vi "HFRR ADV v026 new software.vi"() -> ()   [LabVIEW 2025] (continued)
            n898 = Number To Fractional String(number=w899, width (-)=i16 4, precision (6)=i16 7) -> (F-format string=w905:string)  [unwired: 1 in]
            n899 = Number To Fractional String(number=w901, width (-)=i16 10 ("precision (6)"), precision (6)=i16 7) -> (F-format string=w931:string)  [unwired: 1 in]
            n900 = Concatenate Strings("[CH1]" ("string"), w931, " - 5x Gain" ("string"), "\r") -> (w921:string)
            n901 = Concatenate Strings("[CH2]" ("string"), w922, " - 10x Gain" ("string"), "\r") -> (w920:string)
            n902 = Concatenate Strings("[CH3]" ("string"), w917, " - 20x Gain" ("string"), "\r") -> (w911:string)
            n903 = Concatenate Strings("[CH4]" ("string"), w905, " - 100x Gain" ("string"), "\r") -> (w904:string)
            n904 = String To Path(string="C:\\LAB-IQ\\Image Calibrate v01.dcf") -> (path=w934:path)
            n905 = Concatenate Strings(w921, w920, w911, w904) -> (w919:string)
            n906 = call <vilib>:"Write Characters To File.vi"("append to file? (new file:F)"=FALSE, "character string"=w919, "file path (dialog if empty)"=w934) -> ()  [unwired: 2 in, 1 out]
          }
          frame #2 {
            n907 = String To Path(string="C:\\LAB-IQ\\Image Calibrate v01.dcf") -> (path=w937:path)
            n908 = Open/Create/Replace File ("Open File")(file path (use dialog)=w937) -> (refnum out=w938:refnum<file>)  [unwired: 5 in, 2 out]
            n909 = for {
              N: 4 -> [_]
              tunnel: w938 -> [w944]
              i -> [w940]
              n910 = Read from Text File ("Read File")(file (use dialog)=w944) -> (text=w945:string)  [unwired: 3 in, 3 out]
              n911 = String Subset(string=w945, offset (0)=6, length (rest)=10 ("length (rest)")) -> (substring=w941:string)
              n912 = Fract/Exp String To Number(string=w941) -> (number=w939:dbl)  [unwired: 3 in, 1 out]
              n913 = case shown="3" w940 {
                tunnel: w939 -> [w946 w947 _ w948 _]
                frame 0 {
                  n914 = local write "5x Gain"(w946) -> ()
                }
                frame 1 {
                  n915 = local write "10x Gain"(w947) -> ()
                }
                frame 2 {
                }
                frame 3 {
                  n916 = local write "100x gain"(w948) -> ()
                }
                frame 4, Default {
                }
              }
            }
          }
          frame #3 {
            n917 = call "IMAGE ANALYSIS.vi"("Enum"=POST_ANALYSIS_ENUM."SHOW UI") -> ()  [unwired: 9 in, 2 out]
          }
          frame #4 {
            n918 = Not(x=w951) -> (.not. x?=w950:bool)
            n919 = local write "Save Change"(w950) -> ()
          }
        }
      }
    }
    n920 = case shown="False" w841 {
      tunnel: w840 -> [w867 _]
      frame False {
        n921 = case shown="True" w867 {
          frame False {
          }
          frame True {
            n922 = local read "Set Humidity:"() -> (w871:dbl)
            n923 = local read "Set Humidity:"() -> (w874:dbl)
            n924 = local read "Humidity ( %RH )"() -> (w875:dbl)
            n925 = Subtract(x=w871, y=2.0) -> (x-y=w869:dbl)
            n926 = Add(x=w874, y=2.0) -> (x+y=w870:dbl)
            n927 = In Range and Coerce(upper limit=w870, x=w875, lower limit=w869) -> (In Range?=w868:bool)  [unwired: 1 out]
            n928 = case shown="True" w868 {
              frame False {
              }
              frame True {
                n929 = case shown="True" "Manual Humididty Reached" {
                  selector: "Manual Humididty Reached" -> [_ w878]
                  frame False {
                  }
                  frame True {
                    n930 = Not(x=w878) -> (.not. x?=w877:bool)
                    n931 = local write "Manual Humididty Reached"(w877) -> ()
                    n932 = local read "EVENT LOG"() -> (w880:string)
                    n933 = call "Event Log.vi"("Content"="Target Humidity reached", "EVENT LOG"=w880) -> ("EVENT LOG"=w879:string)  [unwired: 8 in, 1 out]
                    n934 = local write "EVENT LOG"(w879) -> ()
                  }
                }
              }
            }
          }
        }
      }
      frame True {
        n935 = local write "Manual Humididty Reached"(TRUE ("Manual Humididty Reached")) -> ()
      }
    }
    n936 = local read "Cap Live Image"() -> (w861:bool)
    n937 = local read "SCAR MEASURMENT"() -> (w864:enum32{"Auto Scar", "Manual Scar"})
    n938 = Wait (ms)(milliseconds to wait=u32 250) -> ()  [unwired: 1 out]
    n939 = Equal?(x=w864, y=enum32{"Auto Scar", "Manual Scar"}."Manual Scar" ("SCAR MEASURMENT")) -> (x = y?=w862:bool)
    n940 = And(x=w862, y=w861) -> (x .and. y?=w860:bool)
    n941 = case shown="True" w860 {
      selector: w860 -> [_ w1176]
      frame False {
      }
      frame True {
        n942 = stacked-sequence {
          tunnel: [_ _ _ w1191 _] -> _
          tunnel: w1176 -> [_ _ _ _ w1198]
          frame #0 {
            w1177 = 0.0
            n943 = local write "Major Axis"(w1177) -> ()
            n944 = local write "Minor Axis"(w1177) -> ()
            n945 = local write "Average"(w1177) -> ()
          }
          frame #1 {
            n946 = call "CAMERA LIVE FEED FGV.vi"("Enum - Menu"=CAMERA_LIVE_FEED_ENUM."CAMERA MINIMIZE") -> ()  [unwired: 9 in, 2 out]
          }
          frame #2 {
            n947 = local read "FILE 3"() -> (w1185:string)
            n948 = call <vilib>:"Trim Whitespace.vi"("string"="C:\\LAB-IQ\\images\\") -> ("trimmed string"=w1187:string)  [unwired: 1 in]
            n949 = String To Path(string=w1187) -> (path=w1186:path)
            n950 = Concatenate Strings(w1185, ".png" ("string")) -> (w1184:string)
            n951 = Build Path(base path=w1186, name or relative path=w1184) -> (appended path=w1182:path)
            n952 = Path To String(path=w1182) -> (string=w1181:string)
            n953 = call "CAMERA LIVE FEED FGV.vi"("Enum - Menu"=CAMERA_LIVE_FEED_ENUM."CAMERA SAVE", "Image Path"=w1181) -> ("error out"=w1179:errorcluster)  [unwired: 8 in, 1 out]
            n954 = case shown="No Error" w1179 {
              frame No Error {
                n955 = One Button Dialog(message="Image saved successfully") -> ()  [unwired: 1 in, 1 out]
              }
              frame Error {
              }
            }
          }
          frame #3 {
            n956 = call "LIST FILE NAMES.vi"() -> ("error out"=w1193:errorcluster, "filenames"=w1190:string[])  [unwired: 10 in]
            n957 = call "IMAGE ANALYSIS.vi"("Enum"=POST_ANALYSIS_ENUM."SHOW UI", "error in"=w1193) -> ("error out"=w1191:errorcluster)  [unwired: 8 in, 1 out]
            n958 = property on="Test File List :" class="CmbBox"("Strings[]"=w1190) -> ()  [unwired: 2 in, 2 out]
          }
          frame #4 {
            (unwired) T23."Report" ("Main Dashboard Buttons")
            (unwired) T25."Report" ("Main Dashboard Buttons")
            n959 = Not(x=w1198) -> (.not. x?=w1197:bool)
            n960 = local write "Zoom Factore"(0.0 ("Zoom Factore")) -> ()
            n961 = local write "Cap Live Image"(w1197) -> ()
            n962 = local write "Main Tab"(T2."Adv Scar Report" ("Main Tab")) -> ()
            n963 = property on="Cap Live Image" class="Bool (strict)"("BoolText.Text"="Capture Image" ("Boolean Text.Text")) -> ()  [unwired: 2 in, 2 out]
            n964 = local write "Main Dashboard Buttons"(T1."Report" ("Main Dashboard Buttons")) -> ()
          }
        }
      }
    }
    n965 = local read "change Gain"() -> (w844:bool)
    n966 = local read "Back Square"() -> (w843:bool)
    n967 = case shown="True" w844 {
      selector: w844 -> [_ w888]
      frame False {
      }
      frame True {
        n968 = stacked-sequence {
          tunnel: w888 -> [_ w896]
          frame #0 {
            n969 = local read "Actual (µm)"() -> (w892:dbl)
            n970 = local read "Pixel Value"() -> (w891:dbl)
            n971 = local read "Magnification :"() -> (w890:string)
            n972 = Divide(x=w892, y=w891) -> (x/y=w889:dbl)
            n973 = case shown="\"10x\"" w890 {
              tunnel: w889 -> [w893 w894]
              frame "10x" {
                n974 = local write "10x Gain"(w893) -> ()
              }
              frame "5x", Default {
                n975 = local write "5x Gain"(w894) -> ()
              }
            }
          }
          frame #1 {
            n976 = Not(x=w896) -> (.not. x?=w895:bool)
            n977 = local write "change Gain"(w895) -> ()
          }
        }
      }
    }
    n978 = case shown="True" w843 {
      selector: w843 -> [_ w886]
      frame False {
      }
      frame True {
        n979 = Not(x=w886) -> (.not. x?=w885:bool)
        n980 = local write "Back Square"(w885) -> ()
        n981 = local write "Calibration Tab"(enum32{"Measrument", "Calibrate"}."Measrument" ("Calibration Tab")) -> ()
      }
    }
    n982 = local read "Rectangle Tool"() -> (w855:bool)
    n983 = local read "Clear ROI Tool"() -> (w854:bool)
    n984 = local read "Open Image"() -> (w859:bool)
    n985 = local read "line tool"() -> (w856:bool)
    n986 = local read "OUT"() -> (w857:bool)
    n987 = local read "In"() -> (w858:bool)
    n988 = case shown="True" w859 {
      selector: w859 -> [_ w1164]
      tunnel: [w1160 w1166] -> _
      tunnel: w849 -> [w1160 w1165]
      frame False {
      }
      frame True {
        n989 = Not(x=w1164) -> (.not. x?=w1163:bool)
        n990 = local write "Open Image"(w1163) -> ()
        n991 = call "IMAGE ANALYSIS.vi"("Enum"=POST_ANALYSIS_ENUM."HIDE UI", "error in"=w1165) -> ("error out"=w1173:errorcluster)  [unwired: 8 in, 1 out]
        n992 = call "File Dialog"("start path"=path "C:/LAB-IQ/images", "error in"=w1173) -> ("selected path"=w1162:path, "error out"=w1171:errorcluster)  [unwired: 10 in, 2 out]
        "Image path  2" <- w1162
        n993 = call <vilib>:"Clear Errors.vi"("error in (no error)"=w1171) -> ("error out"=w1170:errorcluster)  [unwired: 5 in, 1 out]
        n994 = call "IMAGE ANALYSIS.vi"("Enum"=POST_ANALYSIS_ENUM."OPEN FILE", "error in"=w1170, "File Path"=w1162) -> ("error out"=w1169:errorcluster)  [unwired: 7 in, 1 out]
        n995 = call <vilib>:"Clear Errors.vi"("error in (no error)"=w1169) -> ("error out"=w1168:errorcluster)  [unwired: 5 in, 1 out]
        n996 = call "IMAGE ANALYSIS.vi"("Enum"=POST_ANALYSIS_ENUM."SHOW UI", "error in"=w1168) -> ("error out"=w1166:errorcluster)  [unwired: 8 in, 1 out]
        n997 = local write "Zoom Factore"(100.0 ("Zoom Factore")) -> ()
      }
    }
    n998 = case shown="True" w857 {
      selector: w857 -> [_ w1145]
      tunnel: w849 -> [w1142 w1150]
      tunnel: [w1142 w1144] -> _
      frame False {
      }
      frame True {
        n999 = Not(x=w1145) -> (.not. x?=w1143:bool)
        n1000 = local read "Zoom Factore"() -> (w1148:dbl)
        n1001 = local write "OUT"(w1143) -> ()
        n1002 = call "IMAGE ANALYSIS.vi"("Enum"=POST_ANALYSIS_ENUM."ZOOM OUT", "error in"=w1150) -> ("error out"=w1144:errorcluster)  [unwired: 8 in, 1 out]
        n1003 = Divide(x=w1148, y=1.2) -> (x/y=w1146:dbl)
        n1004 = local write "Zoom Factore"(w1146) -> ()
      }
    }
    n1005 = case shown="True" w858 {
      selector: w858 -> [_ w1154]
      tunnel: w849 -> [w1151 w1159]
      tunnel: [w1151 w1152] -> _
      frame False {
      }
      frame True {
        n1006 = Not(x=w1154) -> (.not. x?=w1153:bool)
        n1007 = local read "Zoom Factore"() -> (w1157:dbl)
        n1008 = local write "In"(w1153) -> ()
        n1009 = call "IMAGE ANALYSIS.vi"("Enum"=POST_ANALYSIS_ENUM."ZOOM IN", "error in"=w1159) -> ("error out"=w1152:errorcluster)  [unwired: 8 in, 1 out]
        n1010 = Multiply(x=w1157, y=1.2) -> (x*y=w1155:dbl)
        n1011 = local write "Zoom Factore"(w1155) -> ()
      }
    }
    n1012 = case shown="True" w854 {
      selector: w854 -> [_ w1126]
      tunnel: w849 -> [w1124 w1128]
      tunnel: [w1124 w1127] -> _
      frame False {
      }
      frame True {
        n1013 = Not(x=w1126) -> (.not. x?=w1125:bool)
        n1014 = local write "Clear ROI Tool"(w1125) -> ()
        n1015 = call "IMAGE ANALYSIS.vi"("Enum"=POST_ANALYSIS_ENUM."CLEAR ROI", "error in"=w1128) -> ("error out"=w1127:errorcluster)  [unwired: 8 in, 1 out]
      }
    }
    n1016 = case shown="True" w856 {
      selector: w856 -> [_ w1138]
      tunnel: w849 -> [w1136 w1141]
      tunnel: [w1136 w1139] -> _
      frame False {
      }
      frame True {
        n1017 = Not(x=w1138) -> (.not. x?=w1137:bool)
        n1018 = local write "line tool"(w1137) -> ()
        n1019 = call "IMAGE ANALYSIS.vi"("Enum"=POST_ANALYSIS_ENUM."DRAW LINE", "error in"=w1141) -> ("error out"=w1139:errorcluster)  [unwired: 8 in, 1 out]
      }
    }
    n1020 = case shown="True" w855 {
      selector: w855 -> [_ w1132]
      tunnel: w849 -> [w1130 w1134]
      tunnel: [w1130 w1133] -> _
      frame False {
      }
      frame True {
        n1021 = Not(x=w1132) -> (.not. x?=w1131:bool)
        n1022 = local write "Rectangle Tool"(w1131) -> ()
        n1023 = call "IMAGE ANALYSIS.vi"("Enum"=POST_ANALYSIS_ENUM."DRAW REC", "error in"=w1134) -> ("error out"=w1133:errorcluster)  [unwired: 8 in, 1 out]
      }
    }
    n1024 = local read "SCAR MEASURMENT"() -> (w842:enum32{"Auto Scar", "Manual Scar"})
    n1025 = local read "Fit to Screen Tool"() -> (w851:bool)
    n1026 = local read "Resize Tool"() -> (w850:bool)
    n1027 = case shown="\"Manual Scar\", Default" w842 {
      frame "Auto Scar" {
        n1028 = property on="Cap Live Image" class="Bool (strict)"("BoolText.Text"="Report" ("Boolean Text.Text")) -> ()  [unwired: 2 in, 2 out]
      }
      frame "Manual Scar", Default {
        n1029 = property on="Cap Live Image" class="Bool (strict)"("BoolText.Text"="Save Image" ("Boolean Text.Text")) -> ()  [unwired: 2 in, 2 out]
      }
    }
    n1030 = local read "ROI Color Tool"() -> (w852:bool)
    n1031 = local read "Pan Tool"() -> (w853:bool)
    n1032 = case shown="True" w853 {
      selector: w853 -> [_ w1120]
      tunnel: w849 -> [w1118 w1122]
      tunnel: [w1118 w1121] -> _
      frame False {
      }
      frame True {
        n1033 = Not(x=w1120) -> (.not. x?=w1119:bool)
        n1034 = call "IMAGE ANALYSIS.vi"("Enum"=POST_ANALYSIS_ENUM."PAN", "error in"=w1122) -> ("error out"=w1121:errorcluster)  [unwired: 8 in, 1 out]
        n1035 = local write "Pan Tool"(w1119) -> ()
      }
    }
    n1036 = case shown="True" w850 {
      selector: w850 -> [_ w1104]
      tunnel: w849 -> [w1099 w1101]
      tunnel: [w1099 w1100] -> _
      frame False {
      }
      frame True {
        n1037 = Not(x=w1104) -> (.not. x?=w1103:bool)
        n1038 = local write "Resize Tool"(w1103) -> ()
        n1039 = call "IMAGE ANALYSIS.vi"("Enum"=POST_ANALYSIS_ENUM."RESIZE MODE", "error in"=w1101) -> ("error out"=w1100:errorcluster)  [unwired: 8 in, 1 out]
      }
    }
    n1040 = case shown="True" w851 {
      selector: w851 -> [_ w1109]
      tunnel: [w1105 w1110] -> _
      tunnel: w849 -> [w1105 w1108]
      frame False {
      }
      frame True {
        n1041 = Not(x=w1109) -> (.not. x?=w1107:bool)
        n1042 = local write "Zoom Factore"(100.0 ("Zoom Factore")) -> ()
        n1043 = local write "Fit to Screen Tool"(w1107) -> ()
        n1044 = call "IMAGE ANALYSIS.vi"("Enum"=POST_ANALYSIS_ENUM."FIT", "error in"=w1108) -> ("error out"=w1110:errorcluster)  [unwired: 8 in, 1 out]
      }
    }
    n1045 = case shown="True" w852 {
      selector: w852 -> [_ w1115]
      tunnel: [w1112 w1116] -> _
      tunnel: w849 -> [w1112 w1113]
      frame False {
      }
      frame True {
        n1046 = Not(x=w1115) -> (.not. x?=w1114:bool)
        n1047 = local write "ROI Color Tool"(w1114) -> ()
        n1048 = call "IMAGE ANALYSIS.vi"("Enum"=POST_ANALYSIS_ENUM."SET ROI COLOR", "error in"=w1113) -> ("error out"=w1116:errorcluster)  [unwired: 8 in, 1 out]
      }
    }
    n1049 = local read "Quit"() -> (w866:bool)
  }
  n1050 = while {
    stop <- w1200 stop-if-true
    n1051 = local read "Image Path"() -> (w1203:path)
    n1052 = local read "Print 3"() -> (w1206:bool)
    n1053 = Equal?(x=w1203, y=path "") -> (x = y?=w1202:bool)
    n1054 = Not(x=w1202) -> (.not. x?=w1201:bool)
    n1055 = property on="Print 3" class="Bool (strict)"("Visible"=w1201) -> ()  [unwired: 2 in, 2 out]
    n1056 = case shown="True" w1206 {
      frame False {
        n1057 = local write "Rd"(TRUE ("Boolean 7")) -> ()
      }
      frame True {
        n1058 = flat-sequence {
          tunnel: [w1246] -> w1214
          tunnel: [w1233] -> w1212
          tunnel: [w1243] -> w1208
          tunnel: w1214 -> [w1255]
          tunnel: [w1255] -> w1213
          tunnel: w1212 -> [w1254]
          tunnel: [w1254] -> w1211
          tunnel: [w1252] -> w1210
          tunnel: [w1251] -> w1209
          tunnel: w1208 -> [w1251]
          tunnel: w1213 -> [w1257]
          tunnel: w1211 -> [w1258]
          tunnel: w1210 -> [_]
          tunnel: w1209 -> [w1256]
          frame #0 {
            n1059 = case shown="True" "Rd" {
              frame False {
              }
              frame True {
                n1060 = while {
                  tunnel: "abcdefABCDEF" ("string 2") -> [w1225]
                  shift-right: [w1223] -> w1217
                  shift-left: "" -> [w1222]
                  i -> [w1232]
                  stop <- w1231 stop-if-true
                  n1061 = Random Number (0-1)() -> (number: 0 to 1=w1226:dbl)
                  n1062 = Multiply(x=w1226, y=62.0) -> (x*y=w1228:dbl)
                  n1063 = Decrement(x="Length 2") -> (x-1=w1221:i16)
                  n1064 = To Word Integer(number=w1228) -> (16bit integer=w1229:i16)
                  n1065 = String Subset(string=w1225, offset (0)=w1229, length (rest)=1 ("length (rest)")) -> (substring=w1224:string)
                  n1066 = Greater Or Equal?(x=w1232, y=w1221) -> (x >= y?=w1231:bool)
                  n1067 = Concatenate Strings(w1224, w1222) -> (w1223:string)
                }
                "String 10" <- w1217
                n1068 = local write "Rd"(FALSE ("Boolean 7")) -> ()
              }
            }
          }
          frame #1 {
            w1244 = "_resized.jpg" ("command line")
            (unwired) ".jpg -resize 320x240 " ("string")
            (unwired) "Choose an Image File" ("prompt")
            # "-resize 1798x425"
            n1069 = local read "Image Path"() -> (w1238:path)
            n1070 = Strip Path(path=w1238) -> (stripped path=w1233:path, name=w1234:string)
            n1071 = Match Pattern(string=w1234, regular expression=".jpg") -> (before substring=→"before substring 2":string, after substring=→"after substring":string)  [unwired: 1 in, 2 out]
            n1072 = Match Pattern(string=w1234, regular expression="\\") -> (before substring=w1240:string)  [unwired: 1 in, 3 out]
            n1073 = Match Pattern(string=w1240, regular expression=".jpg") -> (before substring=w1239:string)  [unwired: 1 in, 3 out]
            n1074 = Concatenate Strings("cmd /c convert " ("string"), w1239, ".jpg -resize 320x240  " ("command line"), w1239, w1244) -> (w1247:string)
            n1075 = call <vilib>:"System Exec.vi"("run minimized? (F)"=TRUE, "wait until completion? (T)"=TRUE, "working directory"=w1233, "command line"=w1247) -> ("error out"=w1246:errorcluster)  [unwired: 4 in, 3 out]
            "error out 2" <- w1246
            n1076 = Concatenate Strings(w1239, w1244) -> (w1243:string)
          }
          frame #2 {
            n1077 = Wait (ms)(milliseconds to wait=u32 2000 ("millisecond timer value")) -> (millisecond timer value=w1252:u32)
          }
          frame #3 {
            n1078 = case shown="No Error" w1257 {
              tunnel: w1258 -> [w1261 _]
              tunnel: w1256 -> [w1259 _]
              frame No Error {
                (unwired) ".jpg" ("string")
                n1079 = Path To String(path=w1261) -> (string=w1265:string)
                n1080 = Concatenate Strings(w1265, "\\" ("string"), w1259) -> (w1264:string)
                n1081 = String To Path(string=w1264) -> (path=w1263:path)
                n1082 = call <vilib>:"Read JPEG File.vi"("path to JPEG file"=w1263) -> ("image data"=w1267:T15)  [unwired: 8 in, 2 out]
                "image data" <- w1267
                n1083 = local write "Print 3"(FALSE ("Print 2")) -> ()
                n1084 = call <vilib>:"Draw Flattened Pixmap.vi"("image data"=w1267) -> ("new picture"=→"new picture":picture)  [unwired: 8 in]
              }
              frame Error {
              }
            }
          }
        }
      }
    }
    n1085 = Wait (ms)(milliseconds to wait=u32 20 ("millisecond timer value")) -> ()  [unwired: 1 out]
    n1086 = local read "Quit"() -> (w1200:bool)
  }
  n1087 = while {
    tunnel: w38 -> [_]
    tunnel: w24 -> [_]
    stop <- w1297 stop-if-true
    # "New Adv Logics"
    n1088 = local read "Main Tab"() -> (w1278:T2)
    n1089 = local read "Main Tab"() -> (w1295:T2)
    n1090 = local read "Sign In"() -> (w1294:bool)
    n1091 = case shown="\"Adv Scar\"" w1278 {
      frame "HOME", Default {
        n1092 = local read "LIVE FEED MIN TEMP"() -> (w1430:bool)
        n1093 = local write "LIVE FEED MAX TEMP"(TRUE ("LIVE FEED MAX TEMP")) -> ()
        n1094 = local read "CAMERA ROI MIN TEMP"() -> (w1428:bool)
        n1095 = case shown="True" w1430 {
          selector: w1430 -> [_ w1437]
          frame False {
          }
          frame True {
            n1096 = Not(x=w1437) -> (.not. x?=w1436:bool)
            n1097 = local write "LIVE FEED MIN TEMP"(w1436) -> ()
            n1098 = call "CAMERA LIVE FEED FGV.vi"("Enum - Menu"=CAMERA_LIVE_FEED_ENUM."CAMERA MINIMIZE") -> ()  [unwired: 9 in, 2 out]
          }
        }
        n1099 = case shown="True" w1428 {
          selector: w1428 -> [_ w1434]
          frame False {
          }
          frame True {
            n1100 = Not(x=w1434) -> (.not. x?=w1433:bool)
            n1101 = local write "CAMERA ROI MIN TEMP"(w1433) -> ()
            n1102 = call "IMAGE ANALYSIS.vi"("Enum"=POST_ANALYSIS_ENUM."MINIMIZE UI") -> ()  [unwired: 9 in, 2 out]
          }
        }
        n1103 = local write "CAMERA ROI MAX TEMP"(TRUE ("CAMERA ROI MAX TEMP")) -> ()
      }
      frame "Test Setup" {
        n1104 = local read "LIVE FEED MIN TEMP"() -> (w1440:bool)
        n1105 = local read "CAMERA ROI MIN TEMP"() -> (w1438:bool)
        n1106 = local write "LIVE FEED MAX TEMP"(TRUE ("LIVE FEED MAX TEMP")) -> ()
        n1107 = case shown="True" w1440 {
          selector: w1440 -> [_ w1447]
          frame False {
          }
          frame True {
            n1108 = Not(x=w1447) -> (.not. x?=w1446:bool)
            n1109 = local write "LIVE FEED MIN TEMP"(w1446) -> ()
            n1110 = call "CAMERA LIVE FEED FGV.vi"("Enum - Menu"=CAMERA_LIVE_FEED_ENUM."CAMERA MINIMIZE") -> ()  [unwired: 9 in, 2 out]
          }
        }
        n1111 = case shown="True" w1438 {
          selector: w1438 -> [_ w1444]
          frame False {
          }
          frame True {
            n1112 = Not(x=w1444) -> (.not. x?=w1443:bool)
            n1113 = local write "CAMERA ROI MIN TEMP"(w1443) -> ()
            n1114 = call "IMAGE ANALYSIS.vi"("Enum"=POST_ANALYSIS_ENUM."MINIMIZE UI") -> ()  [unwired: 9 in, 2 out]
          }
        }
        n1115 = local write "CAMERA ROI MAX TEMP"(TRUE ("CAMERA ROI MAX TEMP")) -> ()
      }
      frame "Acquire" {
        n1116 = local read "LIVE FEED MIN TEMP"() -> (w1450:bool)
        n1117 = local write "LIVE FEED MAX TEMP"(TRUE ("LIVE FEED MAX TEMP")) -> ()
        n1118 = local read "CAMERA ROI MIN TEMP"() -> (w1448:bool)
        n1119 = case shown="True" w1450 {
          selector: w1450 -> [_ w1457]
          frame False {
          }
          frame True {
            n1120 = Not(x=w1457) -> (.not. x?=w1456:bool)
            n1121 = local write "LIVE FEED MIN TEMP"(w1456) -> ()
            n1122 = call "CAMERA LIVE FEED FGV.vi"("Enum - Menu"=CAMERA_LIVE_FEED_ENUM."CAMERA MINIMIZE") -> ()  [unwired: 9 in, 2 out]
          }
        }
        n1123 = case shown="True" w1448 {
          selector: w1448 -> [_ w1454]
          frame False {
          }
          frame True {
            n1124 = Not(x=w1454) -> (.not. x?=w1453:bool)
            n1125 = local write "CAMERA ROI MIN TEMP"(w1453) -> ()
            n1126 = call "IMAGE ANALYSIS.vi"("Enum"=POST_ANALYSIS_ENUM."MINIMIZE UI") -> ()  [unwired: 9 in, 2 out]
          }
        }
        n1127 = local write "CAMERA ROI MAX TEMP"(TRUE ("CAMERA ROI MAX TEMP")) -> ()
      }
      frame "Adv Scar" {
        n1128 = local read "CAMERA ROI MIN TEMP"() -> (w1458:bool)
        n1129 = case shown="True" "LIVE FEED MAX TEMP" {
          selector: "LIVE FEED MAX TEMP" -> [_ w1479]
          frame False {
          }
          frame True {
            n1130 = Not(x=w1479) -> (.not. x?=w1478:bool)
            n1131 = local write "LIVE FEED MAX TEMP"(w1478) -> ()
            n1132 = call "CAMERA LIVE FEED FGV.vi"("Enum - Menu"=CAMERA_LIVE_FEED_ENUM."CAMERA RESTORE") -> ("error out"=w1469:errorcluster)  [unwired: 9 in, 1 out]
            n1133 = Type Cast(type=30, x=0) -> (*(type *) &x=w1473:i32)
            n1134 = Add(x=w1473, y=48) -> (x+y=w1474:i32)
            n1135 = call "CAMERA LIVE FEED FGV.vi"("Enum - Menu"=CAMERA_LIVE_FEED_ENUM."CAMERA MODE SET", "error in (no error)"=w1469, "CAMERA MODE"=w1474) -> ("error out"=w1466:errorcluster)  [unwired: 7 in, 1 out]
            n1136 = call "CAMERA LIVE FEED FGV.vi"("Enum - Menu"=CAMERA_LIVE_FEED_ENUM."CAMERA GRAY", "error in (no error)"=w1466) -> ("error out"=w1465:errorcluster)  [unwired: 8 in, 1 out]
            n1137 = call "LIST FILE NAMES.vi"("error in (no error)"=w1465) -> ("error out"=w1475:errorcluster, "filenames"=w1476:string[])  [unwired: 9 in]
            n1138 = property on="FILE 3" class="CmbBox"(error in=w1475, "Strings[]"=w1476) -> ()  [unwired: 1 in, 2 out]
          }
        }
        n1139 = case shown="True" w1458 {
          selector: w1458 -> [_ w1464]
          frame False {
          }
          frame True {
            n1140 = Not(x=w1464) -> (.not. x?=w1463:bool)
            n1141 = local write "CAMERA ROI MIN TEMP"(w1463) -> ()
            n1142 = call "IMAGE ANALYSIS.vi"("Enum"=POST_ANALYSIS_ENUM."MINIMIZE UI") -> ()  [unwired: 9 in, 2 out]
          }
        }
        n1143 = local write "CAMERA ROI MAX TEMP"(TRUE ("CAMERA ROI MAX TEMP")) -> ()
        "LIVE FEED MIN TEMP" <- TRUE ("LIVE FEED MIN TEMP")
      }
      frame "Adv Scar Report" {
        n1144 = local read "CAMERA ROI MAX TEMP"() -> (w1480:bool)
        n1145 = local read "LIVE FEED MIN TEMP"() -> (w1482:bool)
        n1146 = local write "LIVE FEED MAX TEMP"(TRUE ("LIVE FEED MAX TEMP")) -> ()
        n1147 = case shown="True" w1482 {
          selector: w1482 -> [_ w1491]
          frame False {
          }
          frame True {
            n1148 = Not(x=w1491) -> (.not. x?=w1490:bool)
            n1149 = local write "LIVE FEED MIN TEMP"(w1490) -> ()
            n1150 = call "CAMERA LIVE FEED FGV.vi"("Enum - Menu"=CAMERA_LIVE_FEED_ENUM."CAMERA MINIMIZE") -> ()  [unwired: 9 in, 2 out]
          }
        }
        n1151 = case shown="True" w1480 {
          selector: w1480 -> [_ w1488]
          frame False {
          }
          frame True {
            n1152 = Not(x=w1488) -> (.not. x?=w1486:bool)
            n1153 = local write "CAMERA ROI MAX TEMP"(w1486) -> ()
            n1154 = call "IMAGE ANALYSIS.vi"("Enum"=POST_ANALYSIS_ENUM."SHOW UI") -> ("error out"=w1485:errorcluster)  [unwired: 9 in, 1 out]
            n1155 = call "LIST FILE NAMES.vi"("error in (no error)"=w1485) -> ("filenames"=w1484:string[])  [unwired: 9 in, 1 out]
            n1156 = property on="Test File List :" class="CmbBox"("Strings[]"=w1484) -> ()  [unwired: 2 in, 2 out]
          }
        }
        n1157 = local write "CAMERA ROI MIN TEMP"(TRUE ("CAMERA ROI MIN TEMP")) -> ()
      }
      frame "Compare Files" {
        n1158 = local read "LIVE FEED MIN TEMP"() -> (w1494:bool)
        n1159 = local write "LIVE FEED MAX TEMP"(TRUE ("LIVE FEED MAX TEMP")) -> ()
        n1160 = local read "CAMERA ROI MIN TEMP"() -> (w1492:bool)
        n1161 = case shown="True" w1494 {
          selector: w1494 -> [_ w1501]
          frame False {
          }
          frame True {
            n1162 = Not(x=w1501) -> (.not. x?=w1500:bool)
            n1163 = local write "LIVE FEED MIN TEMP"(w1500) -> ()
            n1164 = call "CAMERA LIVE FEED FGV.vi"("Enum - Menu"=CAMERA_LIVE_FEED_ENUM."CAMERA MINIMIZE") -> ()  [unwired: 9 in, 2 out]
          }
        }
        n1165 = case shown="True" w1492 {
          selector: w1492 -> [_ w1498]
          frame False {
          }
          frame True {
            n1166 = Not(x=w1498) -> (.not. x?=w1497:bool)
            n1167 = local write "CAMERA ROI MIN TEMP"(w1497) -> ()
            n1168 = call "IMAGE ANALYSIS.vi"("Enum"=POST_ANALYSIS_ENUM."MINIMIZE UI") -> ()  [unwired: 9 in, 2 out]
          }
        }
        n1169 = local write "CAMERA ROI MAX TEMP"(TRUE ("CAMERA ROI MAX TEMP")) -> ()
      }
      frame "About" {
        n1170 = local read "LIVE FEED MIN TEMP"() -> (w1504:bool)
        n1171 = local write "LIVE FEED MAX TEMP"(TRUE ("LIVE FEED MAX TEMP")) -> ()
        n1172 = local read "CAMERA ROI MIN TEMP"() -> (w1503:bool)
        n1173 = case shown="True" w1504 {
          selector: w1504 -> [_ w1511]
          frame False {
          }
          frame True {
            n1174 = Not(x=w1511) -> (.not. x?=w1510:bool)
            n1175 = local write "LIVE FEED MIN TEMP"(w1510) -> ()
            n1176 = call "CAMERA LIVE FEED FGV.vi"("Enum - Menu"=CAMERA_LIVE_FEED_ENUM."CAMERA MINIMIZE") -> ()  [unwired: 9 in, 2 out]
          }
        }
        n1177 = case shown="True" w1503 {
          selector: w1503 -> [_ w1508]
          frame False {
          }
          frame True {
            n1178 = Not(x=w1508) -> (.not. x?=w1507:bool)
            n1179 = local write "CAMERA ROI MIN TEMP"(w1507) -> ()
            n1180 = call "IMAGE ANALYSIS.vi"("Enum"=POST_ANALYSIS_ENUM."MINIMIZE UI") -> ()  [unwired: 9 in, 2 out]
          }
        }
        n1181 = local write "CAMERA ROI MAX TEMP"(TRUE ("CAMERA ROI MIN TEMP")) -> ()
      }
      frame "Advance" {
        n1182 = local read "LIVE FEED MIN TEMP"() -> (w1514:bool)
        n1183 = local write "LIVE FEED MAX TEMP"(TRUE ("LIVE FEED MAX TEMP")) -> ()
        n1184 = local read "CAMERA ROI MIN TEMP"() -> (w1512:bool)
        n1185 = case shown="True" w1514 {
          selector: w1514 -> [_ w1521]
          frame False {
          }
          frame True {
            n1186 = Not(x=w1521) -> (.not. x?=w1520:bool)
            n1187 = local write "LIVE FEED MIN TEMP"(w1520) -> ()
            n1188 = call "CAMERA LIVE FEED FGV.vi"("Enum - Menu"=CAMERA_LIVE_FEED_ENUM."CAMERA MINIMIZE") -> ()  [unwired: 9 in, 2 out]
          }
        }
        n1189 = local write "CAMERA ROI MAX TEMP"(TRUE ("CAMERA ROI MAX TEMP")) -> ()
        n1190 = case shown="True" w1512 {
          selector: w1512 -> [_ w1518]
          frame False {
          }
          frame True {
            n1191 = Not(x=w1518) -> (.not. x?=w1517:bool)
            n1192 = local write "CAMERA ROI MIN TEMP"(w1517) -> ()
            n1193 = call "IMAGE ANALYSIS.vi"("Enum"=POST_ANALYSIS_ENUM."MINIMIZE UI") -> ()  [unwired: 9 in, 2 out]
          }
        }
      }
      frame "Mooha" {
        n1194 = local read "LIVE FEED MIN TEMP"() -> (w1524:bool)
        n1195 = local write "LIVE FEED MAX TEMP"(TRUE ("LIVE FEED MAX TEMP")) -> ()
        n1196 = local read "CAMERA ROI MIN TEMP"() -> (w1522:bool)
        n1197 = case shown="True" w1524 {
          selector: w1524 -> [_ w1531]
          frame False {
          }
          frame True {
            n1198 = Not(x=w1531) -> (.not. x?=w1530:bool)
            n1199 = local write "LIVE FEED MIN TEMP"(w1530) -> ()
            n1200 = call "CAMERA LIVE FEED FGV.vi"("Enum - Menu"=CAMERA_LIVE_FEED_ENUM."CAMERA MINIMIZE") -> ()  [unwired: 9 in, 2 out]
          }
        }
        n1201 = local write "CAMERA ROI MAX TEMP"(TRUE ("CAMERA ROI MAX TEMP")) -> ()
        n1202 = case shown="True" w1522 {
          selector: w1522 -> [_ w1528]
          frame False {
          }
          frame True {
            n1203 = Not(x=w1528) -> (.not. x?=w1527:bool)
            n1204 = local write "CAMERA ROI MIN TEMP"(w1527) -> ()
            n1205 = call "IMAGE ANALYSIS.vi"("Enum"=POST_ANALYSIS_ENUM."MINIMIZE UI") -> ()  [unwired: 9 in, 2 out]
          }
        }
      }
    }
    n1206 = local read "Auto Start Test"() -> (w1269:bool)
    n1207 = case shown="True" "sign in temp" {
      frame False {
      }
      frame True {
        w1304 = 1 ("y")
        n1208 = local read "USERNAME"() -> (w1310:string)
        n1209 = local read "USER ID"() -> (w1307:string)
        n1210 = call <vilib>:"Trim Whitespace.vi"("string"=w1310) -> ("trimmed string"=w1309:string)  [unwired: 1 in]
        n1211 = call <vilib>:"Trim Whitespace.vi"("string"=w1307) -> ("trimmed string"=w1308:string)  [unwired: 1 in]
        n1212 = String Length(string=w1309) -> (length=w1306:i32)
        n1213 = String Length(string=w1308) -> (length=w1305:i32)
        n1214 = Greater?(x=w1306, y=w1304) -> (0:w1303:bool)
        n1215 = Greater?(x=w1305, y=w1304) -> (0:w1302:bool)
        n1216 = And(x=w1303, y=w1302) -> (x .and. y?=w1301:bool)
        n1217 = case shown="True" w1301 {
          frame False {
            n1218 = property on="Sign In" class="Bool (strict)"("DisabledEnum"=T18."Disabled" ("Disabled")) -> ()  [unwired: 2 in, 2 out]
          }
          frame True {
            n1219 = property on="Sign In" class="Bool (strict)"("DisabledEnum"=T18."Enabled" ("Disabled")) -> ()  [unwired: 2 in, 2 out]
          }
        }
      }
    }
    n1220 = local read "Air Temperature"() -> (w1286:bool)
    n1221 = local read "Coefficient Of Friction"() -> (w1287:bool)
    n1222 = case shown="False" w1269 {
      frame False {
        n1223 = local read "Auto stop temp"() -> (w1298:bool)
        n1224 = case shown="True" w1298 {
          frame False {
          }
          frame True {
            n1225 = local write "Auto Start Temp"(FALSE ("Auto Start Temp")) -> ()
          }
        }
      }
      frame True {
        "Auto stop temp" <- TRUE ("Auto stop temp")
      }
    }
    n1226 = local read "Humidity"() -> (w1285:bool)
    n1227 = case shown="\"HOME\"" w1295 {
      frame "HOME" {
        n1228 = local write "main tab sub"(enum32{"Page 1", "Page 2"}."Page 1" ("main tab sub")) -> ()
      }
      frame Default {
        n1229 = local write "main tab sub"(enum32{"Page 1", "Page 2"}."Page 2" ("main tab sub")) -> ()
      }
    }
    n1230 = case shown="True" w1294 {
      selector: w1294 -> [_ w1645]
      frame False {
      }
      frame True {
        n1231 = Not(x=w1645) -> (.not. x?=w1644:bool)
        n1232 = local write "Sign In"(w1644) -> ()
        n1233 = local write "Main Dashboard Buttons"(T23."Test Setup" ("Main Dashboard Buttons")) -> ()
      }
    }
    n1234 = case shown="\"Numeric Display\", Default" "Num/Graph" {
      frame "Numeric Display", Default {
        n1235 = property on="Single/Multiple" class="RadioBtnsControl (strict)"("Visible"=FALSE) -> ()  [unwired: 2 in, 2 out]
        n1236 = property on="Single - Graph" class="Ring (strict)"("Visible"=FALSE) -> ()  [unwired: 2 in, 2 out]
        n1237 = local write "Main Tab Display"(T4."Dashboard 1" ("Main Tab Display")) -> ()
      }
      frame "Graph Display" {
        n1238 = property on="Single/Multiple" class="RadioBtnsControl (strict)"("Visible"=TRUE) -> ()  [unwired: 2 in, 2 out]
        n1239 = case shown="\"Multiple\"" "Single/Multiple" {
          frame "Single ", Default {
            n1240 = property on="Single - Graph" class="Ring (strict)"("Visible"=TRUE) -> ()  [unwired: 2 in, 2 out]
            n1241 = local write "Main Tab Display"(T4."Dashboard 3" ("Main Tab Display")) -> ()
          }
          frame "Multiple" {
            n1242 = property on="Single - Graph" class="Ring (strict)"("Visible"=FALSE) -> ()  [unwired: 2 in, 2 out]
            n1243 = local write "Main Tab Display"(T4."Dashboard 2" ("Main Tab Display")) -> ()
          }
        }
      }
    }
    n1244 = local read "Stroke"() -> (w1284:bool)
    n1245 = local read "USERNAME"() -> (w1289:string)
    n1246 = case shown="True" w1287 {
      selector: w1287 -> [_ w1571]
      frame False {
      }
      frame True {
        n1247 = Not(x=w1571) -> (.not. x?=w1570:bool)
        n1248 = local write "Coefficient Of Friction"(w1570) -> ()
        n1249 = local write "Tab Control 2"(T6."Coefficient Of Friction" ("Tab Control 2")) -> ()
      }
    }
    n1250 = case shown="True" w1286 {
      selector: w1286 -> [_ w1568]
      frame False {
      }
      frame True {
        n1251 = Not(x=w1568) -> (.not. x?=w1566:bool)
        n1252 = local write "Air Temperature"(w1566) -> ()
        n1253 = local write "Tab Control 2"(T6."Air Temperature" ("Tab Control 2")) -> ()
      }
    }
    n1254 = case shown="True" w1284 {
      selector: w1284 -> [_ w1562]
      frame False {
      }
      frame True {
        n1255 = Not(x=w1562) -> (.not. x?=w1560:bool)
        n1256 = local write "Stroke"(w1560) -> ()
        n1257 = local write "Tab Control 2"(T6."Stroke" ("Tab Control 2")) -> ()
      }
    }
    n1258 = local write "tested by"(w1289) -> ()
    n1259 = case shown="True" w1285 {
      selector: w1285 -> [_ w1565]
      frame False {
      }
      frame True {
        n1260 = Not(x=w1565) -> (.not. x?=w1563:bool)
        n1261 = local write "Humidity"(w1563) -> ()
        n1262 = local write "Tab Control 2"(T6."Humidity" ("Tab Control 2")) -> ()
      }
    }
    n1263 = case shown="\"Calibration\"" "Main Dashboard Buttons" {
      tunnel: [T2."HOME" ("Main Tab") T2."Test Setup" ("Main Tab") T2."Acquire" ("Main Tab") T2."Adv Scar" ("Main Tab") T2."Adv Scar Report" ("Main Tab") T2."Compare Files" ("Main Tab") T2."Calibration" ("Main Tab") T2."About" ("Main Tab") T2."Advance" ("Main Tab")] -> w1268
      frame "Home", Default {
      }
      frame "Test Setup" {
      }
      frame "Dashboard" {
      }
      frame "Imaging" {
      }
      frame "Report" {
      }
      frame "Analysis" {
      }
      frame "Calibration" {
      }
      frame "About" {
      }
      frame "Advance" {
      }
    }
    n1264 = Wait (ms)(milliseconds to wait=u32 100) -> ()  [unwired: 1 out]
    n1265 = local read "Main Tab Display"() -> (w1288:T4)
    n1266 = local write "Main Tab"(w1268) -> ()
    n1267 = case shown="\"Dashboard 3\"" w1288 {
      frame "Dashboard 1", Default {
        n1268 = property on="Reset Graph" class="Bool (strict)"("Visible"=FALSE) -> ()  [unwired: 2 in, 2 out]
      }
      frame "Dashboard 2" {
        n1269 = property on="Reset Graph" class="Bool (strict)"("Visible"=TRUE) -> ()  [unwired: 2 in, 2 out]
      }
      frame "Dashboard 3" {
        n1270 = property on="Reset Graph" class="Bool (strict)"("Visible"=TRUE) -> ()  [unwired: 2 in, 2 out]
      }
    }
    n1271 = local read "SCAR MEASURMENT"() -> (w1276:enum32{"Auto Scar", "Manual Scar"})
    n1272 = local read "Humidity"() -> (w1290:bool)
    n1273 = local read "Cap Live Image"() -> (w1273:bool)
    n1274 = local read "Sample Temperature"() -> (w1283:bool)
    n1275 = local read "Air Temp vs Humidity"() -> (w1281:bool)
    n1276 = local read "Frequency"() -> (w1282:bool)
    n1277 = case shown="True" w1290 {
      frame False {
        n1278 = local write "Humidity On Command"(TRUE ("Humidity On Command")) -> ()
        n1279 = case shown="True" "Humidity Off Command" {
          selector: "Humidity Off Command" -> [_ w1578]
          frame False {
          }
          frame True {
            n1280 = stacked-sequence {
              frame #0 {
                n1281 = local read "Write UNO"() -> (w1580:string[])
                n1282 = Insert Into Array(array=w1580, new element="R;1" ("new element/subarray")) -> (w1579:string[])  [unwired: 1 in]
                n1283 = local write "Write UNO"(w1579) -> ()
              }
              frame #1 {
                n1284 = Wait (ms)(milliseconds to wait=u32 2000) -> ()  [unwired: 1 out]
              }
              frame #2 {
                n1285 = local read "Write UNO"() -> (w1583:string[])
                n1286 = local read "EVENT LOG"() -> (w1587:string)
                n1287 = call "Event Log.vi"("Content"="Humidity Control Off" ("string"), "EVENT LOG"=w1587) -> ("EVENT LOG"=w1588:string)  [unwired: 8 in, 1 out]
                n1288 = local write "EVENT LOG"(w1588) -> ()
                n1289 = Insert Into Array(array=w1583, new element="R;1" ("new element/subarray")) -> (w1584:string[])  [unwired: 1 in]
                n1290 = local write "Write UNO"(w1584) -> ()
              }
            }
            n1291 = Not(x=w1578) -> (.not. x?=w1577:bool)
            n1292 = local write "Humidity Off Command"(w1577) -> ()
          }
        }
      }
      frame True {
        n1293 = local write "Humidity Off Command"(TRUE ("Humidity Off Command")) -> ()
        n1294 = case shown="True" "Humidity On Command" {
          selector: "Humidity On Command" -> [_ w1592]
          frame False {
          }
          frame True {
            n1295 = stacked-sequence {
              frame #0 {
                n1296 = local read "Set Rh"() -> (w1598:dbl)
                n1297 = local read "Write UNO"() -> (w1593:string[])
                n1298 = Number To Fractional String(number=w1598, precision (6)=i16 2) -> (F-format string=w1599:string)  [unwired: 2 in]
                n1299 = Concatenate Strings("M;" ("new element/subarray"), w1599) -> (w1597:string)
                n1300 = Insert Into Array(array=w1593, new element=w1597) -> (w1594:string[])  [unwired: 1 in]
                n1301 = local write "Write UNO"(w1594) -> ()
              }
              frame #1 {
                n1302 = Wait (ms)(milliseconds to wait=u32 2000) -> ()  [unwired: 1 out]
              }
              frame #2 {
                n1303 = local read "Set Rh"() -> (w1606:dbl)
                n1304 = local read "Write UNO"() -> (w1601:string[])
                n1305 = Number To Fractional String(number=w1606, precision (6)=i16 2) -> (F-format string=w1607:string)  [unwired: 2 in]
                n1306 = Concatenate Strings("M;" ("new element/subarray"), w1607) -> (w1605:string)
                n1307 = Insert Into Array(array=w1601, new element=w1605) -> (w1602:string[])  [unwired: 1 in]
                n1308 = local write "Write UNO"(w1602) -> ()
              }
              frame #3 {
                n1309 = Wait (ms)(milliseconds to wait=u32 1500) -> ()  [unwired: 1 out]
              }
              frame #4 {
                (unwired) "% RH" ("string")
                (unwired) i16 2 ("precision (6)")
                (unwired) "M;" ("new element/subarray")
                n1310 = local read "Set Rh"() -> (w1616:dbl)
                n1311 = local read "Write UNO"() -> (w1609:string[])
                n1312 = Number To Fractional String(number=w1616, precision (6)=i16 2) -> (F-format string=w1613:string)  [unwired: 2 in]
                n1313 = Concatenate Strings("M;" ("new element/subarray"), w1613) -> (w1617:string)
                n1314 = Concatenate Strings("Humidity Set to : " ("string"), w1613, "% RH" ("string")) -> (w1611:string)
                n1315 = Insert Into Array(array=w1609, new element=w1617) -> (w1610:string[])  [unwired: 1 in]
                n1316 = disable-structure shown="Enabled" {
                  frame Enabled {
                    n1317 = local read "EVENT LOG"() -> (w1620:string)
                    n1318 = call "Event Log.vi"("Content"="Humidity Control On", "EVENT LOG"=w1620) -> ("EVENT LOG"=w1621:string)  [unwired: 8 in, 1 out]
                    n1319 = local write "EVENT LOG"(w1621) -> ()
                  }
                  frame Disabled {
                  }
                }
                n1320 = disable-structure shown="Enabled" {
                  disable-tunnel: w1611 -> [_ _]
                  frame Enabled {
                    n1321 = local read "EVENT LOG"() -> (w1623:string)
                    n1322 = call "Event Log.vi"("Content"="Humidity Control On", "EVENT LOG"=w1623) -> ("EVENT LOG"=w1624:string)  [unwired: 8 in, 1 out]
                    n1323 = local write "EVENT LOG"(w1624) -> ()
                  }
                  frame Disabled {
                  }
                }
                n1324 = local write "Write UNO"(w1610) -> ()
              }
            }
            n1325 = Not(x=w1592) -> (.not. x?=w1591:bool)
            n1326 = local write "Humidity On Command"(w1591) -> ()
          }
        }
      }
    }
    n1327 = Equal?(x=w1276, y=enum32{"Auto Scar", "Manual Scar"}."Auto Scar" ("SCAR MEASURMENT")) -> (x = y?=w1272:bool)
    n1328 = local read "TEST STANDARD"() -> (w1279:T3)
    n1329 = And(x=w1273, y=w1272) -> (x .and. y?=w1274:bool)
    n1330 = case shown="True" w1274 {
      selector: w1274 -> [_ w1377]
      tunnel: errorcluster {"status"=FALSE, "code"=0, "source"=""} ("error in (no error) 3") -> [_ w1378]
      frame False {
      }
      frame True {
        n1331 = stacked-sequence {
          tunnel: w1378 -> [_ _ _ _ _ _ _ w1426]
          tunnel: w1377 -> [_ _ _ _ _ w1407 _ _]
          frame #0 {
            n1332 = call "CAMERA LIVE FEED FGV.vi"("Enum - Menu"=CAMERA_LIVE_FEED_ENUM."CAMERA MINIMIZE") -> ()  [unwired: 9 in, 2 out]
          }
          frame #1 {
            n1333 = property on="Auto Scar Check  2" class="Clust (strict)"("Visible"=TRUE) -> ()  [unwired: 2 in, 2 out]
          }
          frame #2 {
            n1334 = String To Path(string="C:\\LAB-IQ\\Image Calibrate v01.dcf") -> (path=w1383:path)
            n1335 = Open/Create/Replace File ("Open File")(file path (use dialog)=w1383) -> (refnum out=w1384:refnum<file>)  [unwired: 5 in, 2 out]
            n1336 = for {
              N: 4 -> [_]
              tunnel: w1384 -> [w1390]
              i -> [w1386]
              n1337 = Read from Text File ("Read File")(file (use dialog)=w1390) -> (text=w1391:string)  [unwired: 3 in, 3 out]
              n1338 = String Subset(string=w1391, offset (0)=6, length (rest)=10 ("length (rest)")) -> (substring=w1387:string)
              n1339 = Fract/Exp String To Number(string=w1387) -> (number=w1385:dbl)  [unwired: 3 in, 1 out]
              n1340 = case shown="0" w1386 {
                tunnel: w1385 -> [w1392 w1393 _ w1394 _]
                frame 0 {
                  "5x Gain" <- w1392
                }
                frame 1 {
                  "10x Gain" <- w1393
                }
                frame 2 {
                }
                frame 3 {
                  "100x gain" <- w1394
                }
                frame 4, Default {
                }
              }
            }
          }
          frame #3 {
            n1341 = local read "FILE 3"() -> (w1400:string)
            n1342 = call <vilib>:"Trim Whitespace.vi"("string"="C:\\LAB-IQ\\images\\") -> ("trimmed string"=w1402:string)  [unwired: 1 in]
            n1343 = String To Path(string=w1402) -> (path=w1401:path)
            n1344 = Concatenate Strings(w1400, ".png" ("string")) -> (w1399:string)
            n1345 = Build Path(base path=w1401, name or relative path=w1399) -> (appended path=w1397:path)
            "Image path" <- w1397
            n1346 = Path To String(path=w1397) -> (string=w1396:string)
            n1347 = call "CAMERA LIVE FEED FGV.vi"("Enum - Menu"=CAMERA_LIVE_FEED_ENUM."CAMERA SAVE", "Image Path"=w1396) -> ()  [unwired: 8 in, 2 out]
          }
          frame #4 {
            n1348 = One Button Dialog(message="Image saved successfully") -> ()  [unwired: 1 in, 1 out]
          }
          frame #5 {
            n1349 = local read "TEST STANDARD"() -> (w1406:T3)
            n1350 = local read "Magnification len live scar"() -> (w1418:string)
            n1351 = Not(x=w1407) -> (.not. x?=w1408:bool)
            n1352 = local write "Cap Live Image"(w1408) -> ()
            n1353 = case shown="\"ISO 12156\"" w1406 {
              tunnel: ["ASTM D6079" "ISO 12156"] -> w1405
              frame "ASTM D6079", Default {
              }
              frame "ISO 12156" {
              }
            }
            n1354 = case shown="\"5x\", Default" w1418 {
              tunnel: [w1421 w1422] -> w1417
              frame "5x", Default {
                n1355 = local read "5x Gain"() -> (w1421:dbl)
              }
              frame "10x" {
                # "5x"
                n1356 = local read "10x Gain"() -> (w1422:dbl)
              }
            }
            n1357 = local read "Image path"() -> (w1416:path)
            n1358 = local read "FILE 3"() -> (w1409:string)
            n1359 = call "EDGE DETCTION.vi"("GAIN VALUE"=w1417, "Image Path"=w1416) -> ("error out"=w1415:errorcluster, "return value"=w1414:cluster{string, string, dbl, dbl, dbl})  [unwired: 8 in]
            n1360 = Bundle By Name(cluster=T24 {"File Name"="", "Test Method"="", "Operator"="", "Fuel Description"="", "Date and time"=""} ("Main Ref"), "File Name"=w1409, "Test Method"=w1405) -> (w1410:T24)
            n1361 = call "duf file read.vi"("error in (no error)"=w1415, "Main Ref"=w1410) -> ("error out"=w1413:errorcluster, "Main Ref 2"=w1411:T24)  [unwired: 8 in]
            n1362 = call "EDGE DETECTION REPORT.vi"("error in (no error)"=w1413, "return value 2"=w1414, "Main Ref"=w1411) -> ()  [unwired: 8 in, 1 out]
          }
          frame #6 {
            n1363 = property on="Auto Scar Check  2" class="Clust (strict)"("Visible"=FALSE) -> ()  [unwired: 2 in, 2 out]
          }
          frame #7 {
            n1364 = call "CAMERA LIVE FEED FGV.vi"("Enum - Menu"=CAMERA_LIVE_FEED_ENUM."CAMERA MINIMIZE", "error in (no error)"=w1426) -> ()  [unwired: 8 in, 2 out]
            n1365 = local write "Main Dashboard Buttons"(T1."Home" ("Main Dashboard Buttons")) -> ()
            n1366 = local write "Main Tab"(T2."HOME" ("Main Tab")) -> ()
          }
        }
      }
    }
    n1367 = local read "Heater Button"() -> (w1280:bool)
    n1368 = case shown="True" w1282 {
      selector: w1282 -> [_ w1556]
      frame False {
      }
      frame True {
        n1369 = Not(x=w1556) -> (.not. x?=w1554:bool)
        n1370 = local write "Frequency"(w1554) -> ()
        n1371 = local write "Tab Control 2"(T6."Frequency" ("Tab Control 2")) -> ()
      }
    }
    n1372 = case shown="True" w1281 {
      selector: w1281 -> [_ w1553]
      frame False {
      }
      frame True {
        n1373 = Not(x=w1553) -> (.not. x?=w1551:bool)
        n1374 = local write "Air Temp vs Humidity"(w1551) -> ()
        n1375 = local write "Tab Control 2"(T6."Air Temp vs Rh" ("Tab Control 2")) -> ()
      }
    }
    n1376 = case shown="True" w1283 {
      selector: w1283 -> [_ w1559]
      frame False {
      }
      frame True {
        n1377 = Not(x=w1559) -> (.not. x?=w1557:bool)
        n1378 = local write "Sample Temperature"(w1557) -> ()
        n1379 = local write "Tab Control 2"(T6."Sample Temperature" ("Tab Control 2")) -> ()
      }
    }
    n1380 = case shown="\"Custom\"" w1279 {
      frame "ASTM D6079", Default {
        w1532 = "ASTM D6079 TEST CONDITIONS" ("Standard 2")
        n1381 = local write "Standard 2"(w1532) -> ()
        n1382 = local write "Standard"(w1532) -> ()
      }
      frame "ISO 12156" {
        w1533 = "ISO 12156 TEST CONDITIONS" ("Standard 2")
        n1383 = local write "Standard 2"(w1533) -> ()
        n1384 = local write "Standard"(w1533) -> ()
      }
      frame "CEC F-096-A-06" {
        w1534 = "CEC F-096-A-06 TEST CONDITIONS" ("Standard 2")
        n1385 = local write "Standard 2"(w1534) -> ()
        n1386 = local write "Standard"(w1534) -> ()
      }
      frame "Custom" {
        w1535 = "CUSTOM TEST CONDITIONS" ("Standard 2")
        n1387 = local write "Standard 2"(w1535) -> ()
        n1388 = local write "Standard"(w1535) -> ()
      }
    }
    n1389 = case shown="True" w1280 {
      frame False {
        n1390 = local write "Temperature On Command"(TRUE ("Temperature On Command")) -> ()
        n1391 = case shown="True" "Temperature Off Command" {
          selector: "Temperature Off Command" -> [_ w1539]
          frame False {
          }
          frame True {
            n1392 = Not(x=w1539) -> (.not. x?=w1538:bool)
            n1393 = local read "EVENT LOG"() -> (w1542:string)
            n1394 = local write "Temperature Off Command"(w1538) -> ()
            n1395 = call "Event Log.vi"("Content"="Heater Off", "EVENT LOG"=w1542) -> ("EVENT LOG"=w1541:string)  [unwired: 8 in, 1 out]
            n1396 = local write "EVENT LOG"(w1541) -> ()
          }
        }
      }
      frame True {
        n1397 = local write "Temperature Off Command"(TRUE ("Temperature Off Command")) -> ()
        n1398 = case shown="True" "Temperature On Command" {
          selector: "Temperature On Command" -> [_ w1546]
          frame False {
          }
          frame True {
            n1399 = Not(x=w1546) -> (.not. x?=w1545:bool)
            n1400 = local write "Temperature On Command"(w1545) -> ()
            n1401 = disable-structure shown="Enabled" {
              disable-tunnel: "Heater On" -> [w1548 _]
              frame Enabled {
                n1402 = local read "EVENT LOG"() -> (w1549:string)
                n1403 = call "Event Log.vi"("Content"=w1548, "EVENT LOG"=w1549) -> ("EVENT LOG"=w1550:string)  [unwired: 8 in, 1 out]
                n1404 = local write "EVENT LOG"(w1550) -> ()
              }
              frame Disabled {
              }
            }
          }
        }
      }
    }
    n1405 = local read "Main Tab"() -> (w1271:T2)
    n1406 = case shown="\"About\"" w1271 {
      frame "HOME", Default {
        w1313 = T18."Enabled" ("Disabled")
        n1407 = local read "Service Password enable"() -> (w1315:bool)
        n1408 = property on="Imaging" class="Bool (strict)"("DisabledEnum"=w1313) -> ()  [unwired: 2 in, 2 out]
        n1409 = property on="Dashboard" class="Bool (strict)"("DisabledEnum"=w1313) -> ()  [unwired: 2 in, 2 out]
        n1410 = property on="Test Setup" class="Bool (strict)"("DisabledEnum"=w1313) -> ()  [unwired: 2 in, 2 out]
        n1411 = property on="Analysis" class="Bool (strict)"("DisabledEnum"=w1313) -> ()  [unwired: 2 in, 2 out]
        n1412 = property on="Home" class="Bool (strict)"("DisabledEnum"=w1313) -> ()  [unwired: 2 in, 2 out]
        n1413 = property on="Report" class="Bool (strict)"("DisabledEnum"=w1313) -> ()  [unwired: 2 in, 2 out]
        n1414 = property on="Main Dashboard Buttons" class="RadioBtnsControl (strict)"("DisabledEnum"=w1313) -> ()  [unwired: 2 in, 2 out]
        n1415 = property on="Calibration" class="Bool (strict)"("DisabledEnum"=w1313) -> ()  [unwired: 2 in, 2 out]
        n1416 = case shown="True" w1315 {
          tunnel: [T18."Disabled" ("Disabled") T18."Enabled" ("Disabled")] -> w1314
          frame False {
          }
          frame True {
          }
        }
        n1417 = property on="About" class="Bool (strict)"("DisabledEnum"=w1314) -> ()  [unwired: 2 in, 2 out]
      }
      frame "Test Setup" {
        w1320 = T18."Enabled" ("Disabled")
        n1418 = local read "Service Password enable"() -> (w1319:bool)
        n1419 = property on="Dashboard" class="Bool (strict)"("DisabledEnum"=T18."Disabled" ("Disabled")) -> ()  [unwired: 2 in, 2 out]
        n1420 = property on="Imaging" class="Bool (strict)"("DisabledEnum"=w1320) -> ()  [unwired: 2 in, 2 out]
        n1421 = property on="Analysis" class="Bool (strict)"("DisabledEnum"=w1320) -> ()  [unwired: 2 in, 2 out]
        n1422 = property on="Home" class="Bool (strict)"("DisabledEnum"=w1320) -> ()  [unwired: 2 in, 2 out]
        n1423 = property on="Report" class="Bool (strict)"("DisabledEnum"=w1320) -> ()  [unwired: 2 in, 2 out]
        n1424 = property on="Test Setup" class="Bool (strict)"("DisabledEnum"=w1320) -> ()  [unwired: 2 in, 2 out]
        n1425 = case shown="True" w1319 {
          tunnel: [T18."Disabled" ("Disabled") T18."Enabled" ("Disabled")] -> w1318
          frame False {
          }
          frame True {
          }
        }
        n1426 = property on="About" class="Bool (strict)"("DisabledEnum"=w1318) -> ()  [unwired: 2 in, 2 out]
      }
      frame "Adv Scar" {
        w1327 = T18."Enabled" ("Disabled")
        n1427 = property on="Dashboard" class="Bool (strict)"("DisabledEnum"=T18."Disabled" ("Disabled")) -> ()  [unwired: 2 in, 2 out]
        n1428 = property on="Imaging" class="Bool (strict)"("DisabledEnum"=w1327) -> ()  [unwired: 2 in, 2 out]
        n1429 = property on="Analysis" class="Bool (strict)"("DisabledEnum"=w1327) -> ()  [unwired: 2 in, 2 out]
        n1430 = property on="Home" class="Bool (strict)"("DisabledEnum"=w1327) -> ()  [unwired: 2 in, 2 out]
        n1431 = property on="Report" class="Bool (strict)"("DisabledEnum"=w1327) -> ()  [unwired: 2 in, 2 out]
        n1432 = property on="Test Setup" class="Bool (strict)"("DisabledEnum"=w1327) -> ()  [unwired: 2 in, 2 out]
        n1433 = local read "Service Password enable"() -> (w1325:bool)
        n1434 = case shown="True" w1325 {
          tunnel: [T18."Disabled" ("Disabled") T18."Enabled" ("Disabled")] -> w1324
          frame False {
          }
          frame True {
          }
        }
        n1435 = property on="About" class="Bool (strict)"("DisabledEnum"=w1324) -> ()  [unwired: 2 in, 2 out]
      }
      frame "Calibration" {
        w1330 = T18."Enabled" ("Disabled")
        n1436 = property on="Dashboard" class="Bool (strict)"("DisabledEnum"=T18."Disabled" ("Disabled")) -> ()  [unwired: 2 in, 2 out]
        n1437 = property on="Imaging" class="Bool (strict)"("DisabledEnum"=w1330) -> ()  [unwired: 2 in, 2 out]
        n1438 = property on="Analysis" class="Bool (strict)"("DisabledEnum"=w1330) -> ()  [unwired: 2 in, 2 out]
        n1439 = property on="Home" class="Bool (strict)"("DisabledEnum"=w1330) -> ()  [unwired: 2 in, 2 out]
        n1440 = property on="Report" class="Bool (strict)"("DisabledEnum"=w1330) -> ()  [unwired: 2 in, 2 out]
        n1441 = property on="Test Setup" class="Bool (strict)"("DisabledEnum"=w1330) -> ()  [unwired: 2 in, 2 out]
        n1442 = local read "Service Password enable"() -> (w1332:bool)
        n1443 = property on="Calibration" class="Bool (strict)"("DisabledEnum"=w1330) -> ()  [unwired: 2 in, 2 out]
        n1444 = case shown="True" w1332 {
          tunnel: [T18."Disabled" ("Disabled") T18."Enabled" ("Disabled")] -> w1331
          frame False {
          }
          frame True {
          }
        }
        n1445 = property on="About" class="Bool (strict)"("DisabledEnum"=w1331) -> ()  [unwired: 2 in, 2 out]
      }
      frame "Adv Scar Report" {
        w1338 = T18."Enabled" ("Disabled")
        n1446 = property on="Dashboard" class="Bool (strict)"("DisabledEnum"=T18."Disabled" ("Disabled")) -> ()  [unwired: 2 in, 2 out]
        n1447 = property on="Imaging" class="Bool (strict)"("DisabledEnum"=w1338) -> ()  [unwired: 2 in, 2 out]
        n1448 = property on="Analysis" class="Bool (strict)"("DisabledEnum"=w1338) -> ()  [unwired: 2 in, 2 out]
        n1449 = property on="Home" class="Bool (strict)"("DisabledEnum"=w1338) -> ()  [unwired: 2 in, 2 out]
        n1450 = property on="Report" class="Bool (strict)"("DisabledEnum"=w1338) -> ()  [unwired: 2 in, 2 out]
        n1451 = property on="Test Setup" class="Bool (strict)"("DisabledEnum"=w1338) -> ()  [unwired: 2 in, 2 out]
        n1452 = local read "Service Password enable"() -> (w1337:bool)
        n1453 = case shown="True" w1337 {
          tunnel: [T18."Disabled" ("Disabled") T18."Enabled" ("Disabled")] -> w1336
          frame False {
          }
          frame True {
          }
        }
        n1454 = property on="About" class="Bool (strict)"("DisabledEnum"=w1336) -> ()  [unwired: 2 in, 2 out]
      }
      frame "Compare Files" {
        w1344 = T18."Enabled" ("Disabled")
        n1455 = local read "Service Password enable"() -> (w1343:bool)
        n1456 = property on="Dashboard" class="Bool (strict)"("DisabledEnum"=T18."Disabled" ("Disabled")) -> ()  [unwired: 2 in, 2 out]
        n1457 = property on="Imaging" class="Bool (strict)"("DisabledEnum"=w1344) -> ()  [unwired: 2 in, 2 out]
        n1458 = property on="Analysis" class="Bool (strict)"("DisabledEnum"=w1344) -> ()  [unwired: 2 in, 2 out]
        n1459 = property on="Home" class="Bool (strict)"("DisabledEnum"=w1344) -> ()  [unwired: 2 in, 2 out]
        n1460 = property on="Report" class="Bool (strict)"("DisabledEnum"=w1344) -> ()  [unwired: 2 in, 2 out]
        n1461 = property on="Test Setup" class="Bool (strict)"("DisabledEnum"=w1344) -> ()  [unwired: 2 in, 2 out]
        n1462 = case shown="True" w1343 {
          tunnel: [T18."Disabled" ("Disabled") T18."Enabled" ("Disabled")] -> w1342
          frame False {
          }
          frame True {
          }
        }
        n1463 = property on="About" class="Bool (strict)"("DisabledEnum"=w1342) -> ()  [unwired: 2 in, 2 out]
      }
      frame "Acquire" {
        n1464 = local read "Service Password enable"() -> (w1349:bool)
        n1465 = property on="Test Setup" class="Bool (strict)"("DisabledEnum"=T18."Disabled" ("Disabled")) -> ()  [unwired: 2 in, 2 out]
        n1466 = local read "Auto Start Test"() -> (w1351:bool)
        n1467 = local read "RUN"() -> (w1353:bool)
        n1468 = case shown="True" w1349 {
          tunnel: [T18."Disabled" ("Disabled") T18."Enabled" ("Disabled")] -> w1350
          frame False {
          }
          frame True {
          }
        }
        n1469 = Or(x=w1353, y=w1351) -> (x .or. y?=w1352:bool)
        n1470 = case shown="True" w1352 {
          tunnel: [T18."Enabled" ("Disabled") T18."Disabled" ("Disabled")] -> w1348
          frame False {
          }
          frame True {
          }
        }
        n1471 = property on="About" class="Bool (strict)"("DisabledEnum"=w1350) -> ()  [unwired: 2 in, 2 out]
        n1472 = property on="Imaging" class="Bool (strict)"("DisabledEnum"=w1348) -> ()  [unwired: 2 in, 2 out]
